vi "NIIE_Glyph_MouseDown.vi"(6 "Double Click":bool, 8 "Error":errorcluster, 9 "Coords":T5, 10 "CtlRef":refnum<vi>, 11 "Data":T1={"Class"={"Ants"=refnum, "Layer"=refnum, "Templates"=refnum, "Icon"=refnum, "Glyph"=refnum, "Settings"=refnum, "Tools"=refnum}, "Ref"={"Add Layer"=refnum, "Remove Layer"=refnum, "Line Text"=[], "Body Text Spec"=refnum, "DNL_Font"=refnum, "glyph path str"=refnum, "templates path str"=refnum, "Arrow Up"=refnum, "Arrow Down"=refnum, "IE VI Ref"=refnum, "Glyphs tree"=refnum, "Templates tree"=refnum, "Layer Icon Text"=refnum, "Layer Template"=refnum, "Clipboard"=refnum, "BW icon in"=refnum, "Color icon in"=refnum, "Layer Clust"=refnum, "Body Text"=refnum, "DNL_Framework Templates"=refnum, "Search Templates"=refnum, "TextMarker"=refnum, "Tab Control"=refnum, "Search Glyphs"=refnum, "Line Color"=refnum, "DNL_Glyphs []"=refnum, "Fill Color"=refnum, "Tools"=refnum, "Glyphs tree"=refnum, "Icon"=refnum, "Preview"=refnum, "Ants"=refnum, "Terminals"=refnum, "menu reference"=refnum, "LayerNames"=[], "GlyphLoadAnimation"=refnum, "TemplateLoadAnimation"=refnum, "refreshGlyphs"=refnum, "refreshTemplates"=refnum}, "Support"={"AntsRect"={"left"=0, "top"=0, "right"=0, "bottom"=0}, "Mouse Move Coords"={"Horizontal"=0, "Vertical"=0}, "Mouse Down Coords"={"Horizontal"=0, "Vertical"=0}, "Temp Coord"={"Horizontal"=0, "Vertical"=0}, "Action"=enum."Default", "Edge Color"=4914962, "Fill Color"=16860, "Mouse Down?"=FALSE, "Draft Mode?"=FALSE, "Temp Icon"=bytes[3102], "CTRL Pressed"=FALSE, "Move Selection?"=FALSE, "AntsRect Orig"={"left"=0, "top"=0, "right"=0, "bottom"=0}, "Text"="", "TM Set?"=FALSE, "Mouse inside icon?"=FALSE, "Tool (old value)"=0, "Pencil Move Color"=0, "Swap Colors?"=FALSE, "Shift pressed?"=FALSE}}) -> (0 "Error Out":errorcluster, 3 "Data Out":T1={"Class"={"Ants"=refnum, "Layer"=refnum, "Templates"=refnum, "Icon"=refnum, "Glyph"=refnum, "Settings"=refnum, "Tools"=refnum}, "Ref"={"Add Layer"=refnum, "Remove Layer"=refnum, "Line Text"=[], "Body Text Spec"=refnum, "DNL_Font"=refnum, "glyph path str"=refnum, "templates path str"=refnum, "Arrow Up"=refnum, "Arrow Down"=refnum, "IE VI Ref"=refnum, "Glyphs tree"=refnum, "Templates tree"=refnum, "Layer Icon Text"=refnum, "Layer Template"=refnum, "Clipboard"=refnum, "BW icon in"=refnum, "Color icon in"=refnum, "Layer Clust"=refnum, "Body Text"=refnum, "DNL_Framework Templates"=refnum, "Search Templates"=refnum, "TextMarker"=refnum, "Tab Control"=refnum, "Search Glyphs"=refnum, "Line Color"=refnum, "DNL_Glyphs []"=refnum, "Fill Color"=refnum, "Tools"=refnum, "Glyphs tree"=refnum, "Icon"=refnum, "Preview"=refnum, "Ants"=refnum, "Terminals"=refnum, "menu reference"=refnum, "LayerNames"=[], "GlyphLoadAnimation"=refnum, "TemplateLoadAnimation"=refnum, "refreshGlyphs"=refnum, "refreshTemplates"=refnum}, "Support"={"AntsRect"={"left"=0, "top"=0, "right"=0, "bottom"=0}, "Mouse Move Coords"={"Horizontal"=0, "Vertical"=0}, "Mouse Down Coords"={"Horizontal"=0, "Vertical"=0}, "Temp Coord"={"Horizontal"=0, "Vertical"=0}, "Action"=enum."Default", "Edge Color"=4914962, "Fill Color"=16860, "Mouse Down?"=FALSE, "Draft Mode?"=FALSE, "Temp Icon"=bytes[3102], "CTRL Pressed"=FALSE, "Move Selection?"=FALSE, "AntsRect Orig"={"left"=0, "top"=0, "right"=0, "bottom"=0}, "Text"="", "TM Set?"=FALSE, "Mouse inside icon?"=FALSE, "Tool (old value)"=0, "Pencil Move Color"=0, "Swap Colors?"=FALSE, "Shift pressed?"=FALSE}})   [LabVIEW 2021]
uses:
  <vilib>/Utility/miscctls.llb/LVPoint32TypeDef.ctl
  Controls/IE Data.ctl
  Class/Ants/Ants.lvclass
  Class/FakedArray/FakedArray.lvclass
  Class/Icon Library/Glyph.lvclass
  Class/Settings/Settings.lvclass
  Class/Tools/Tools Paint.lvclass
  vi.lib/LabVIEW Icon API/lv_icon/Classes/Icon/Icon.lvclass
  Controls/IE Classes.ctl
  Controls/References Cluster.ctl
  Controls/SupportClass.ctl
  Controls/ENUM_SupportClass_Action.ctl
  vi.lib/LabVIEW Icon API/lv_icon/Controls/IEColor.ctl
  MB CORE/TypeDefs/Cluster_Path&Icon.ctl
  MB CORE/TypeDefs/Cluster_Button Draw Tools.ctl
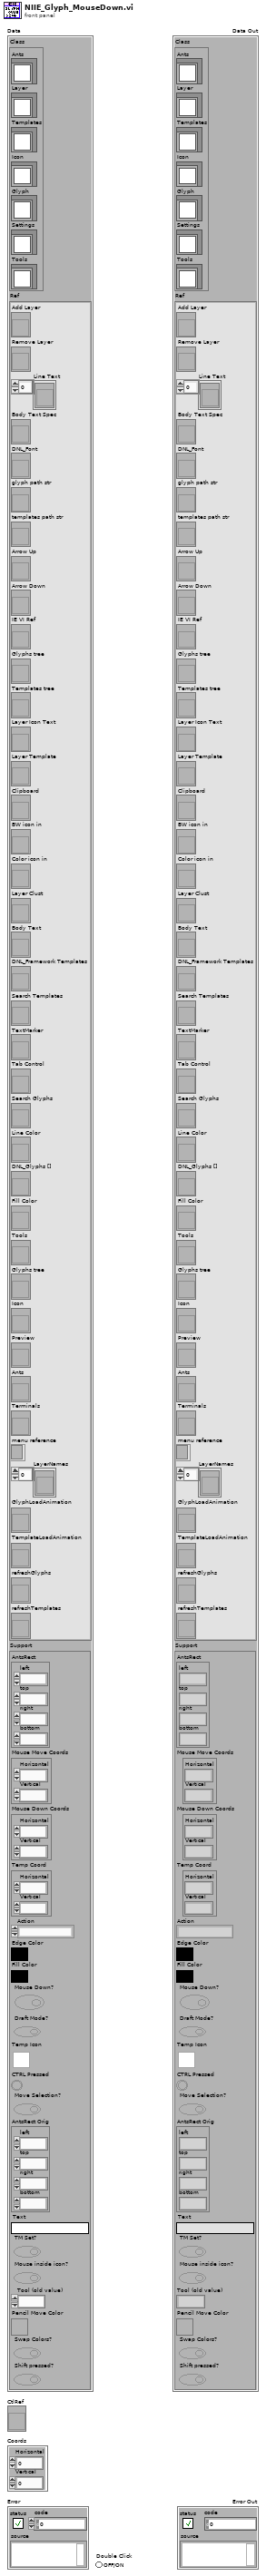
[diagram p1: front panel]
types:
  T1 = typedef "IE Data.ctl" = cluster{"Class":T2, "Ref":T3, "Support":T4}
  T2 = typedef "IE Classes.ctl" = cluster{"Ants":refnum<class "Ants.lvclass">, "Layer":refnum<class "FakedArray.lvclass">, "Templates":refnum<class "FakedArray.lvclass">, "Icon":refnum<class "Icon.lvclass">, "Glyph":refnum<class "Glyph.lvclass">, "Settings":refnum<class "Settings.lvclass">, "Tools":refnum<class "Tools Paint.lvclass">}
  T3 = typedef "References Cluster.ctl" = cluster{"Add Layer":refnum<vi>, "Remove Layer":refnum<vi>, "Line Text":refnum<vi>[], "Body Text Spec":refnum<vi>, "DNL_Font":refnum<vi>, "glyph path str":refnum<vi>, "templates path str":refnum<vi>, "Arrow Up":refnum<vi>, "Arrow Down":refnum<vi>, "IE VI Ref":refnum<vi>, "Glyphs tree":refnum<vi>, "Templates tree":refnum<vi>, "Layer Icon Text":refnum<vi>, "Layer Template":refnum<vi>, "Clipboard":refnum<vi>, "BW icon in":refnum<vi>, "Color icon in":refnum<vi>, "Layer Clust":refnum<vi>, "Body Text":refnum<vi>, "DNL_Framework Templates":refnum<vi>, "Search Templates":refnum<vi>, "TextMarker":refnum<vi>, "Tab Control":refnum<vi>, "Search Glyphs":refnum<vi>, "Line Color":refnum<vi>, "DNL_Glyphs []":refnum<vi>, "Fill Color":refnum<vi>, "Tools":refnum<vi>, "Glyphs tree":refnum<vi>, "Icon":refnum<vi>, "Preview":refnum<vi>, "Ants":refnum<vi>, "Terminals":refnum<vi>, "menu reference":refnum<k9>, "LayerNames":refnum<vi>[], "GlyphLoadAnimation":refnum<vi>, "TemplateLoadAnimation":refnum<vi>, "refreshGlyphs":refnum<vi>, "refreshTemplates":refnum<vi>}
  T4 = typedef "SupportClass.ctl" = cluster{"AntsRect":cluster{"left":i16, "top":i16, "right":i16, "bottom":i16}, "Mouse Move Coords":T5, "Mouse Down Coords":T5, "Temp Coord":T5, "Action":T6, "Edge Color":T7, "Fill Color":T7, "Mouse Down?":bool, "Draft Mode?":bool, "Temp Icon":picture, "CTRL Pressed":bool, "Move Selection?":bool, "AntsRect Orig":cluster{"left":i16, "top":i16, "right":i16, "bottom":i16}, "Text":string, "TM Set?":bool, "Mouse inside icon?":bool, "Tool (old value)":u32, "Pencil Move Color":u32, "Swap Colors?":bool, "Shift pressed?":bool}
  T5 = typedef "LVPoint32TypeDef.ctl" = cluster{"Horizontal":i32, "Vertical":i32}
  T6 = typedef "ENUM_SupportClass_Action.ctl" = enum16{"Default", "Move Selection", "Glyph Library", "Tool"}
  T7 = typedef "IEColor.ctl" = u32
  T8 = typedef "Cluster_Path&Icon.ctl" = cluster{"Rectangle":cluster{"left":i16, "top":i16, "right":i16, "bottom":i16}, "Path":path, "Image":picture, "Filter":string, "FileName":string}
  T9 = typedef "Cluster_Button Draw Tools.ctl" = enum32{"Pencil", "Line", "Dropper", "Fill", "Rectangle", "Filled Rectangle", "Ellipse", "Filled Ellipse", "Eraser", "Text", "Select", "Move"}
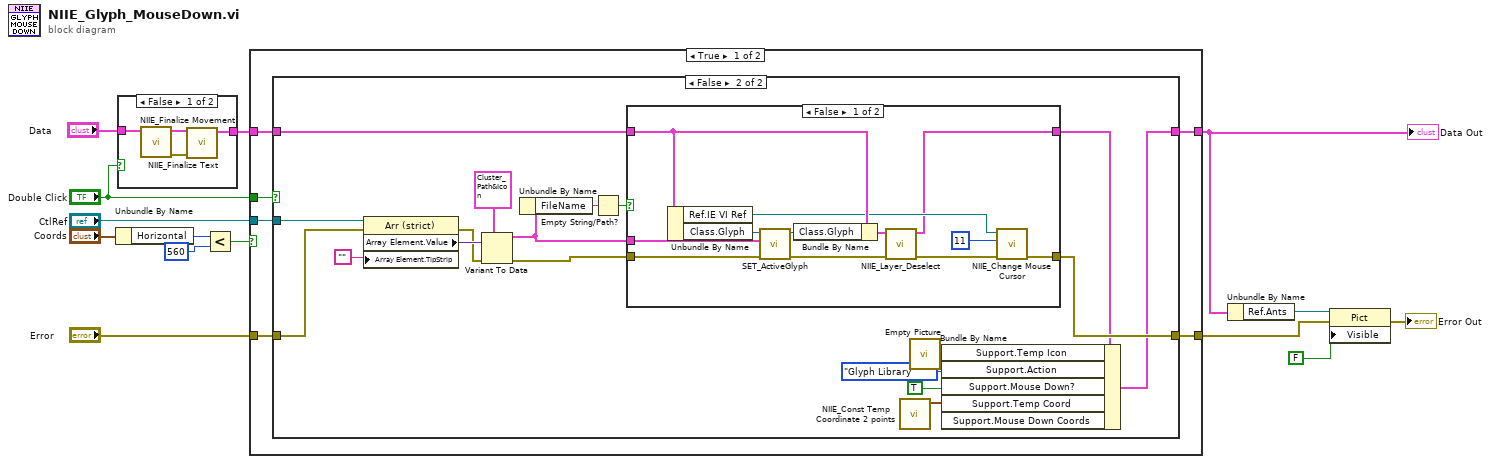
[diagram p0: block diagram]
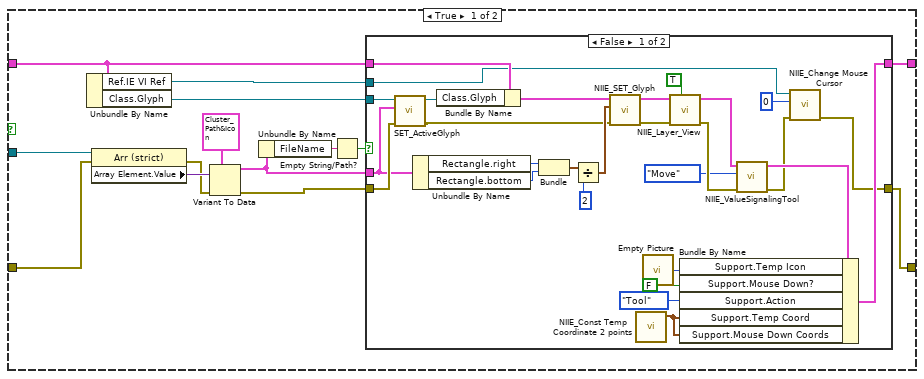
[diagram p3: hidden frame]
diagram:
  n1 = Unbundle By Name("Coords") -> ("Horizontal"=w6:i32)
  n2 = case shown="False" "Double Click" {
    tunnel: "Data" -> [w17 w19]
    tunnel: [w15 w19] -> w4
    frame False {
      n3 = call "NIIE_Finalize Movement.vi"("Data"=w17) -> ("Error Out"=w18:errorcluster, "Data Out"=w16:T1)  [unwired: 2 in, 7 out]
      n4 = call "NIIE_Finalize Text.vi"("Error"=w18, "Data"=w16) -> ("Data Out"=w15:T1)  [unwired: 9 out]
    }
    frame True {
    }
  }
  n5 = Less?(x=w6, y=560 ("x")) -> (x < y?=w8:bool)
  n6 = case shown="True" w8 {
    tunnel: "CtlRef" -> [w25 _]
    tunnel: "Error" -> [w24 w103]
    tunnel: [w23 w103] -> w1
    tunnel: "Double Click" -> [w22 _]
    tunnel: w4 -> [w21 w102]
    tunnel: [w20 w102] -> w2
    frame True {
      n7 = case shown="False" w22 {
        tunnel: w25 -> [w39 w87]
        tunnel: w24 -> [w34 w83]
        tunnel: [w29 w77] -> w23
        tunnel: w21 -> [w32 w75]
        tunnel: [w31 w73] -> w20
        frame True {
          n8 = Unbundle By Name(w32) -> ("Ref.IE VI Ref"=w30:refnum<vi>, "Class.Glyph"=w33:refnum<class "Glyph.lvclass">)
          n9 = property class="Arr (strict)"(reference=w39, error in=w34) -> (error out=w37:errorcluster, "Array Element.Value"=w38:variant)  [unwired: 1 out]
          n10 = Variant To Data(error in=w37, type=T8 {"Rectangle"={"left"=0, "top"=0, "right"=0, "bottom"=0}, "Path"=path "", "Image"=bytes[0], "Filter"="", "FileName"=""} ("Path and Icon"), Variant=w38) -> (data=w27:T8, error out=w35:errorcluster)
          n11 = Unbundle By Name(w27) -> ("FileName"=w28:string)
          n12 = Empty String/Path?(string/path=w28) -> (empty?=w26:bool)
          n13 = case shown="False" w26 {
            tunnel: w35 -> [w67 w68]
            tunnel: w33 -> [w54 _]
            tunnel: w32 -> [w51 w69]
            tunnel: [w50 w69] -> w31
            tunnel: w30 -> [w43 _]
            tunnel: [w41 w68] -> w29
            tunnel: w27 -> [w40 _]
            frame False {
              n14 = call-dynamic "SET_ActiveGlyph.vi"("Error"=w67, "Active Glyph"=w40, "Glyph"=w54) -> ("Error Out"=w52:errorcluster, "Glyph Out"=w53:refnum<class "Glyph.lvclass">)  [unwired: 7 out]
              n15 = Unbundle By Name(w40) -> ("Rectangle.right"=w66:i16, "Rectangle.bottom"=w65:i16)
              n16 = Bundle By Name(cluster=w51, "Class.Glyph"=w53) -> (w49:T1)
              n17 = Bundle("right"=w66, "bottom"=w65) -> (w64:cluster{"right":i16, "bottom":i16})  [unwired: 1 out]
              n18 = Divide(x=w64, y=2) -> (x/y=w62:cluster{"right":dbl, "bottom":dbl})
              n19 = call "NIIE_SET_Glyph.vi"("Error"=w52, "Coordinates"=w62, "Data"=w49) -> ("Error Out"=w56:errorcluster, "Data Out"=w48:T1)  [unwired: 7 out]
              n20 = call "NIIE_Const Temp Coordinate 2 points.vi"() -> ("Const Temp Coordinate"=w58:T5)  [unwired: 11 out]
              n21 = call "Empty Picture"() -> ("empty picture"=w59:picture)
              n22 = call "NIIE_Layer_View.vi"("Add To Undo?"=TRUE ("Add to Undo?"), "Error"=w56, "Data"=w48) -> ("Error Out"=w55:errorcluster, "Data Out"=w46:T1)  [unwired: 2 in, 5 out]
              n23 = call "NIIE_ValueSignalingTool.vi"("Error"=w55, "Tools"=Cluster_Button_Draw_Tools."Move", "Data"=w46) -> ("Error Out"=w42:errorcluster, "Data Out"=w45:T1)  [unwired: 7 out]
              n24 = Bundle By Name(cluster=w45, "Support.Temp Icon"=w59, "Support.Mouse Down?"=FALSE ("Mouse Down?"), "Support.Action"=ENUM_SupportClass_Action."Tool" ("Action"), "Support.Temp Coord"=w58, "Support.Mouse Down Coords"=w58) -> (w50:T1)
              n25 = call "NIIE_Change Mouse Cursor.vi"("error in (no error)"=w42, "icon"=u16 0, "VI reference (current VI)"=w43) -> ("error out"=w41:errorcluster)  [unwired: 8 out]
            }
            frame True {
            }
          }
        }
        frame False {
          n26 = property class="Arr (strict)"(reference=w87, error in=w83, "Array Element.TipStrip"="") -> (error out=w85:errorcluster, "Array Element.Value"=w86:variant)  [unwired: 1 out]
          n27 = Variant To Data(error in=w85, type=T8 {"Rectangle"={"left"=0, "top"=0, "right"=0, "bottom"=0}, "Path"=path "", "Image"=bytes[0], "Filter"="", "FileName"=""} ("Path and Icon"), Variant=w86) -> (data=w72:T8, error out=w76:errorcluster)
          n28 = Unbundle By Name(w72) -> ("FileName"=w70:string)
          n29 = Empty String/Path?(string/path=w70) -> (empty?=w71:bool)
          n30 = case shown="False" w71 {
            tunnel: [w98 w101] -> w77
            tunnel: w76 -> [w97 w101]
            tunnel: w75 -> [w95 w100]
            tunnel: [w89 w100] -> w74
            tunnel: w72 -> [w88 _]
            frame False {
              n31 = Unbundle By Name(w95) -> ("Ref.IE VI Ref"=w94:refnum<vi>, "Class.Glyph"=w92:refnum<class "Glyph.lvclass">)
              n32 = call-dynamic "SET_ActiveGlyph.vi"("Error"=w97, "Active Glyph"=w88, "Glyph"=w92) -> ("Error Out"=w91:errorcluster, "Glyph Out"=w93:refnum<class "Glyph.lvclass">)  [unwired: 7 out]
              n33 = Bundle By Name(cluster=w95, "Class.Glyph"=w93) -> (w90:T1)
              n34 = call "NIIE_Layer_Deselect.vi"("Error"=w91, "Data"=w90) -> ("Error Out"=w99:errorcluster, "Data Out"=w89:T1)  [unwired: 8 out]
              n35 = call "NIIE_Change Mouse Cursor.vi"("error in (no error)"=w99, "icon"=u16 11, "VI reference (current VI)"=w94) -> ("error out"=w98:errorcluster)  [unwired: 8 out]
            }
            frame True {
            }
          }
          n36 = call "NIIE_Const Temp Coordinate 2 points.vi"() -> ("Const Temp Coordinate"=w79:T5)  [unwired: 11 out]
          n37 = call "Empty Picture"() -> ("empty picture"=w80:picture)
          n38 = Bundle By Name(cluster=w74, "Support.Temp Icon"=w80, "Support.Action"=ENUM_SupportClass_Action."Glyph Library" ("Action"), "Support.Mouse Down?"=TRUE ("Mouse Down?"), "Support.Temp Coord"=w79, "Support.Mouse Down Coords"=w79) -> (w73:T1)
        }
      }
    }
    frame False {
    }
  }
  "Data Out" <- w2
  n39 = Unbundle By Name(w2) -> ("Ref.Ants"=w9:refnum<vi>)
  n40 = property class="Pict"(reference=w9, error in=w1, "Visible"=FALSE) -> (error out=→"Error Out":errorcluster)  [unwired: 1 out]
